vi "ProcessImData.vi"(7 "StackSize":cluster{"nX":u32, "nY":u32, "nZ":u32}, 9 "NumChans":u32, 10 "StartingNum":i32, 11 "Data":i32[](array[numeric])) -> (3 "output array":i32[][](array[numeric]))   [LabVIEW 2012]
panel:
  out "size(s)":i32[](array[numeric])
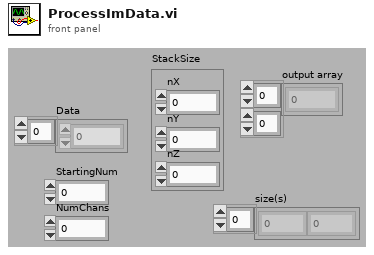
[diagram p1: front panel]
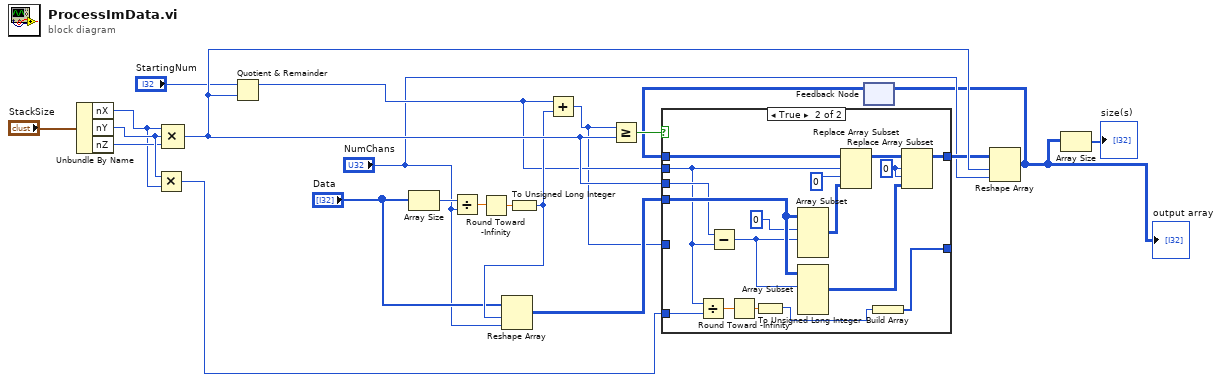
[diagram p0: block diagram]
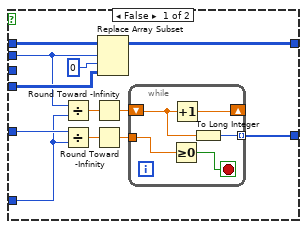
[diagram p2: hidden frame]
diagram:
  n1 = Unbundle By Name("StackSize") -> ("nX"=w5:u32, "nY"=w9:u32, "nZ"=w8:u32)
  n2 = Multiply(x=w9, y=w5) -> (x*y=w7:u32)
  n3 = Compound Arithmetic op=MULTIPLY(w5, w9, w8) -> (w21:u32)
  n4 = Quotient & Remainder(x="StartingNum", y=w21) -> (x-y*floor(x/y)=w14:u32)  [unwired: 1 out]
  n5 = Array Size(array="Data") -> (size(s)=w20:i32)
  n6 = Divide(x=w20, y="NumChans") -> (x/y=w19:dbl)
  n7 = Round Toward -Infinity(1:w19) -> (0:w18:dbl)
  n8 = To Unsigned Long Integer(number=w18) -> (unsigned 32bit integer=w16:u32)
  n9 = Reshape Array("Data", w16, "NumChans") -> (w13:i32[][])
  n10 = Add(x=w14, y=w16) -> (x+y=w6:u32)
  n11 = Greater Or Equal?(x=w6, y=w21) -> (x >= y?=w15:bool)
  n12 = feedback #1() -> (w11:i32[][])  [unwired: 1 in]
  n13 = case shown="True" w15 {
    tunnel: w11 -> [w33 w54]
    tunnel: w14 -> [w29 w43]
    tunnel: w13 -> [w32 w50]
    tunnel: [w31 w52] -> w12
    tunnel: w21 -> [_ w46]
    tunnel: w7 -> [w27 w42]
    tunnel: w6 -> [w28 _]
    tunnel: [w22 w39] -> _
    frame False {
      n14 = Divide(x=w29, y=w27) -> (x/y=w26:dbl)
      n15 = Divide(x=w28, y=w27) -> (x/y=w25:dbl)
      n16 = Round Toward -Infinity(1:w26) -> (0:w24:dbl)
      n17 = Round Toward -Infinity(1:w25) -> (0:w23:dbl)
      n18 = Replace Array Subset(array=w33, new element=w32, index (row)=w29, index (col)=0 ("disabled index (col)")) -> (w31:i32[][])
      n19 = while {
        shift-right: [w38] -> _
        shift-left: w24 -> [w34]
        tunnel: [w35] -> w22 mode=indexing
        tunnel: w23 -> [w37]
        stop <- w36 stop-if-true
        n20 = Greater Or Equal To 0?(x=w37) -> (x >= 0?=w36:bool)
        n21 = Increment(x=w34) -> (x+1=w38:dbl)
        n22 = To Long Integer(number=w34) -> (32bit integer=w35:i32)
      }
    }
    frame True {
      w51 = 0 ("index (row)")
      n23 = Divide(x=w43, y=w42) -> (x/y=w44:dbl)
      n24 = Subtract(x=w46, y=w43) -> (x-y=w45:u32)
      n25 = Round Toward -Infinity(1:w44) -> (0:w41:dbl)
      n26 = To Unsigned Long Integer(number=w41) -> (unsigned 32bit integer=w40:u32)
      n27 = Array Subset(array=w50, index (row)=0 ("index"), length (row)=w45) -> (w49:i32[][])  [unwired: 2 in]
      n28 = Array Subset(array=w50, index (row)=w45) -> (w48:i32[][])  [unwired: 3 in]
      n29 = Replace Array Subset(array=w54, new element=w49, index (row)=w43, index (col)=0 ("disabled index (col)")) -> (w53:i32[][])
      n30 = Build Array(w40) -> (w39:u32[])
      n31 = Replace Array Subset(array=w53, new element=w48, index (row)=w51, index (col)=w51) -> (w52:i32[][])
    }
  }
  n32 = Reshape Array(w12, w21, "NumChans") -> (w1:i32[][])
  "output array" <- w1
  n33 = feedback-in #1(w1) -> ()
  n34 = Array Size(array=w1) -> (size(s)=→"size(s)":i32[])
